vi "Multiples_of_3_or_5_Solution.vi"(4 "Maximum":i32) -> (0 "Sum":i32, 2 "Multiples":i32[](array[numeric]))   [LabVIEW 2013]
panel:
  # "Multiples of 3 or 5\n\nIf we list all the natural numbers below 10 that are multiples of 3 or 5, we get 3, 5, 6 and 9. \nThe sum of these multiples is 23. \n\nCreate a VI that takes one numeric input representing the maximum number and generates an \narray of all multiples of 3 or 5 that are strictly less than that number as well as the sum of all of \nthe multiples."
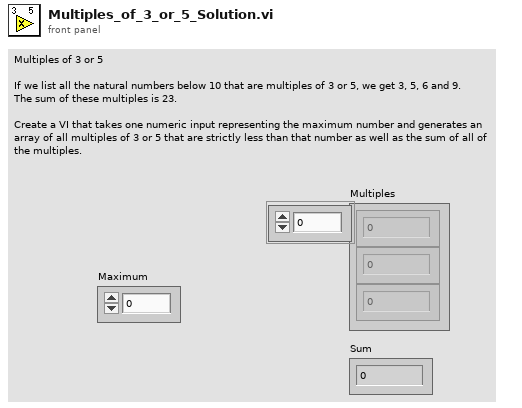
[diagram p1: front panel]
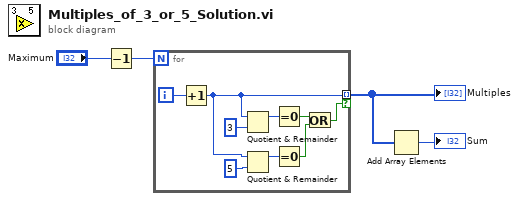
[diagram p0: block diagram]
diagram:
  n1 = Decrement(x="Maximum") -> (x-1=w1:i32)
  n2 = for {
    N: w1 -> [_]
    tunnel: [w5] -> w4 mode=indexing if=w7
    i -> [w6]
    n3 = Increment(x=w6) -> (x+1=w5:i32)
    n4 = Quotient & Remainder(x=w5, y=3) -> (x-y*floor(x/y)=w10:i32)  [unwired: 1 out]
    n5 = Quotient & Remainder(x=w5, y=5) -> (x-y*floor(x/y)=w11:i32)  [unwired: 1 out]
    n6 = Equal To 0?(x=w10) -> (x = 0?=w9:bool)
    n7 = Equal To 0?(x=w11) -> (x = 0?=w8:bool)
    n8 = Or(x=w9, y=w8) -> (x .or. y?=w7:bool)
  }
  "Multiples" <- w4
  n9 = Add Array Elements(numeric array=w4) -> (sum=→"Sum":i32)
